vi "Create Report Queue.vi"(8 "error in":errorcluster, 11 "Base Software in":refnum<class "Base Software.lvclass">) -> (0 "error out":errorcluster, 3 "Base Software out":refnum<class "Base Software.lvclass">)   [LabVIEW 2019, in "Base Software.lvlib" / "Main.lvlib" / "Base Software.lvclass"]
uses:
  Project/Base Software.lvclass
  C:/Users/Public/Documents/Development/builds/Engine/Engine.lvlibp/Project/Engine.lvclass
  builds/Engine/Engine.lvlibp/Accessors/Write Report Queue.vi
  builds/Tools/QDMH.lvlibp/QDMH.lvclass
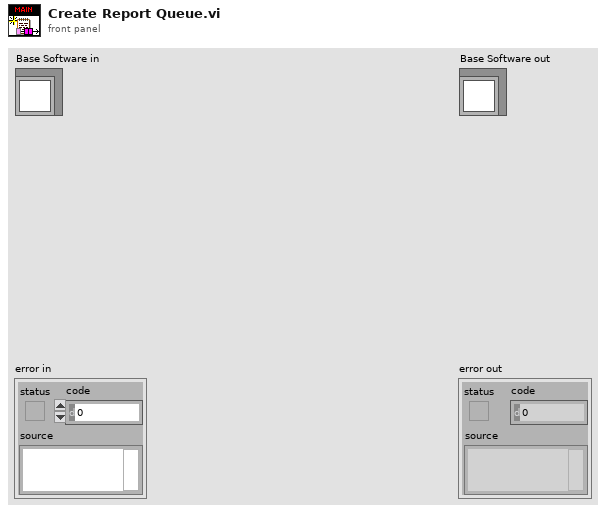
[diagram p1: front panel]
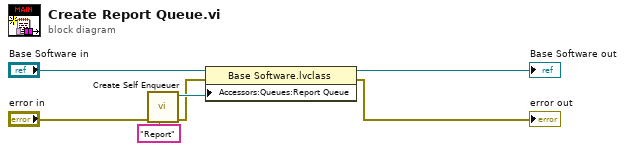
[diagram p0: block diagram]
diagram:
  n1 = call "Create Self Enqueuer.vi"("Name"="Report", "error in"="error in") -> ("error out"=w1:errorcluster, "QDMH out"=w4:refnum<class "QDMH.lvclass">)  [unwired: 8 in]
  n2 = property class="Base Software.lvclass"(reference="Base Software in", error in=w1, "Accessors:Queues:Report Queue"=w4) -> (reference out=→"Base Software out":refnum<class "Base Software.lvclass">, error out=→"error out":errorcluster)
